vi "Teardown.vi"(8 "Error in":errorcluster, 9 "Unhandled Msgs":refnum<class "Msg.lvclass">[](array[class]), 10 "Lifecycle":T1, 11 "TEMPLATE Actor in":refnum<class "TEMPLATE Actor.lvclass">) -> (3 "TEMPLATE Actor out":refnum<class "TEMPLATE Actor.lvclass">)   [LabVIEW 2025, in "_Template.lvlib" / "Templates.lvlib" / "TEMPLATE Actor.lvlib" / "TEMPLATE Actor.lvclass"]
uses:
  TEMPLATE Actor.lvclass
  jettl/jettl/Actor/Lifecycle.ctl
  jettl/jettl/Msg/Msg.lvclass
  TEMPLATE Actor.lvclass/TEMPLATE Actor.ctl
  jettl/jettl/Actor/Actor/Actor.lvclass
  jettl/jettl/Actor/Actor.lvlib
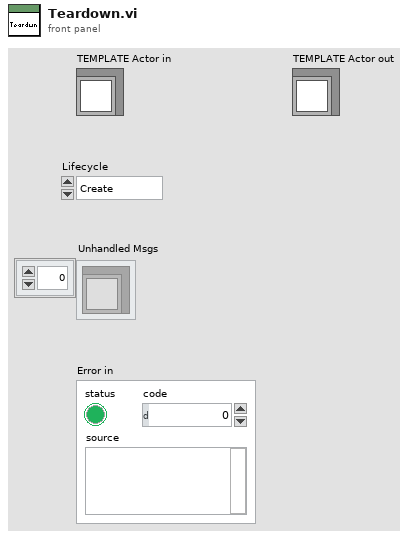
[diagram p1: front panel]
types:
  T1 = typedef "jettl.lvlib/Actor.lvlib/Lifecycle.ctl" = enum16{"Create", "Destroy"}
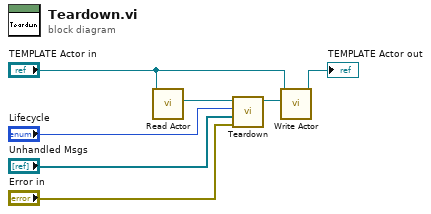
[diagram p0: block diagram]
diagram:
  n1 = call-dynamic "Read Actor.vi"("TEMPLATE Actor in"="TEMPLATE Actor in") -> ("Actor"=w4:refnum<class "Actor.lvclass">)  [unwired: 10 in]
  n2 = call-dynamic "Teardown.vi"("Error in"="Error in", "Unhandled Msgs"="Unhandled Msgs", "Lifecycle"="Lifecycle", "Actor in"=w4) -> ("Actor out"=w2:refnum<class "Actor.lvclass">)  [unwired: 7 in]
  n3 = call-dynamic "Write Actor.vi"("Actor"=w2, "TEMPLATE Actor in"="TEMPLATE Actor in") -> ("TEMPLATE Actor out"=→"TEMPLATE Actor out":refnum<class "TEMPLATE Actor.lvclass">)  [unwired: 9 in]
